vi "Upd MFC Calibrated Gas.vi"(8 "error in (no error)":errorcluster, 10 "MFC Calibrated Gas":string, 11 "FC2901 in":refnum<class "FC2901.lvclass">) -> (0 "error out":errorcluster, 3 "FC2901 out":refnum<class "FC2901.lvclass">)   [LabVIEW 2021, in "FC2901.lvclass"]
uses:
  FC2901.lvclass
  FC2901.lvclass/FC2901.ctl
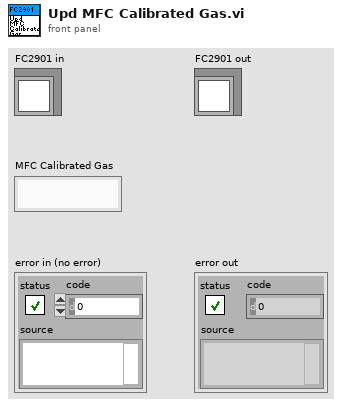
[diagram p1: front panel]
types:
  T1 = typedef "C100L.lvclass/GCF Data.ctl" = map{string, dbl}
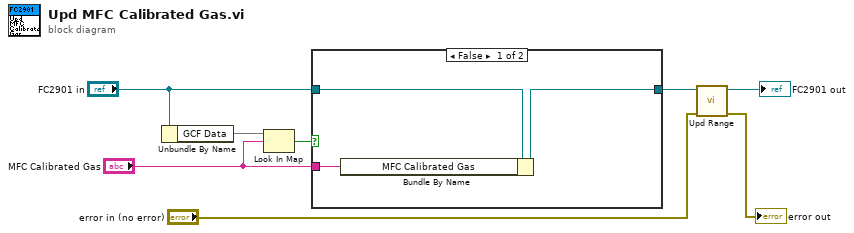
[diagram p0: block diagram]
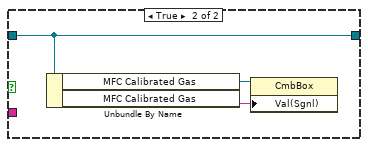
[diagram p2: hidden frame]
diagram:
  n1 = Unbundle By Name("FC2901 in") -> ("GCF Data"=w5:T1)
  n2 = Look In Map(map=w5, key="MFC Calibrated Gas") -> (key not found?=w4:bool)  [unwired: 1 in, 1 out]
  n3 = case shown="False" w4 {
    tunnel: "FC2901 in" -> [w11 w12]
    tunnel: [w10 w12] -> w2
    tunnel: "MFC Calibrated Gas" -> [w9 _]
    frame False {
      n4 = Bundle By Name(cluster=w11, "MFC Calibrated Gas"=w9) -> (w10:refnum<class "FC2901.lvclass">)
    }
    frame True {
      n5 = Unbundle By Name(w12) -> ("MFC Calibrated Gas"=w14:refnum<vi>, "MFC Calibrated Gas"=w13:string)
      n6 = property class="CmbBox"(reference=w14, "Val(Sgnl)"=w13) -> ()  [unwired: 1 in, 2 out]
    }
  }
  n7 = call "Upd Range.vi"("error in (no error)"="error in (no error)", "C100L in"=w2) -> ("error out"=→"error out":errorcluster, "C100L out"=→"FC2901 out":refnum<class "FC2901.lvclass">)  [unwired: 8 in]
